vi "Driver Feedback Loop.vi"   [LabVIEW 2019]
uses:
  Shoot/Shooter Mode Type Def.ctl
  Shoot/Shoot Global.vi
  Vanna/Vanna Global.vi
  Vanna/Vanna Mode Type Def.ctl
  Drive/Drive Global.vi
  Drive/Drive Mode Typedef.ctl
types:
  T1 = typedef "WPI_MotorControlDeviceRef.ctl" = cluster{"DeviceStatus":errorcluster, "Type":T2, "PWM":cluster{"PWM Channel":T3, "DeadBand":T4}, "CAN":cluster{"Device Number":u8, "SetOutput VI Ref":variant, "GetOutput VI Ref":variant, "Enable VI Ref":variant, "Disable VI Ref":variant, "Data":variant}, "Invert":bool, "DIO PWM":cluster{"PWM \"Enable\" Channel":T3, "DIOChannel":T5, "PWM Rate":dbl}}
  T2 = typedef "WPI_MotorControlType.ctl" = enum16{"PWM", "CAN", "DIO PWM"}
  T3 = typedef "FPGA_DIOPWMChannel.ctl" = enum8{"PWM 0", "PWM 1", "PWM 2", "PWM 3", "PWM 4", "PWM 5", "PWM 6", "PWM 7", "PWM 8", "PWM 9", "PWM MXP 0", "PWM MXP 1", "PWM MXP 2", "PWM MXP 3", "PWM MXP 4", "PWM MXP 5", "PWM MXP 6", "PWM MXP 7", "PWM MXP 8", "PWM MXP 9", "Invalid"}
  T4 = typedef "WPI_PWMDeadband.ctl" = cluster{"Name":string, "maxPositivePwm":i32, "minPositivePwm":i32, "centerPwm":i32, "maxNegativePwm":i32, "minNegativePwm":i32, "angularRange":u16}
  T5 = typedef "FPGA_DIOChannel.ctl" = enum8{"DIO 0", "DIO 1", "DIO 2", "DIO 3", "DIO 4", "DIO 5", "DIO 6", "DIO 7", "DIO 8", "DIO 9", "DIO MXP 0", "DIO MXP 1", "DIO MXP 2", "DIO MXP 3", "DIO MXP 4", "DIO MXP 5", "DIO MXP 6", "DIO MXP 7", "DIO MXP 8", "DIO MXP 9", "DIO MXP 10", "DIO MXP 11", "DIO MXP 12", "DIO MXP 13", "DIO MXP 14", "DIO MXP 15", "SPI Port CS1", "SPI Port CS2", "SPI Port CS3", "SPI Port MISO", "SPI Port MOSI", "Invalid"}
  T6 = typedef "WPI_JoystickDevRef.ctl" = cluster{"Device":T7}
  T7 = typedef "WPI_JoystickDeviceEnum.ctl" = enum16{"USB 0", "USB 1", "USB 2", "USB 3", "USB 4", "USB 5"}
  T8 = typedef "Shooter Mode Type Def.ctl" = enum16{"Disabled", "Raw Throttle", "Preset Velocity Control", "Vision-based Velocity Control"}
  T9 = typedef "Drive Mode Typedef.ctl" = enum16{"Disabled", "Auto-align", "Drive Distance", "Turn to angle", "Driver"}
  T10 = typedef "Vanna Mode Type Def.ctl" = enum16{"Disabled", "Raw Throttle", "Rotation Control", "Position Control"}
  T11 = typedef "Vanna Command Type Def.ctl" = cluster{"Vanna Mode":T10, "Throttle (%)":dbl, "Timestamp (ms)":dbl}
  T12 = typedef "Drive Command Typedef.ctl" = cluster{"Drive Mode":T9, "LeftValue(%)/ relative Distance[ft]":dbl, "Right Motor Value(%)/ absolute angle (deg)":dbl, "Timestamp (ms)":dbl}
  T13 = typedef "Shooter Command Type Def.ctl" = cluster{"Shooter Mode":T8, "Throttle (%)/ Vision-based\nSetpoint (RPM)":dbl, "Shooter Preset speeds (RPM)":T14, "Timestamp (ms)":dbl}
  T14 = typedef "Shooter Preset speeds Type Def.ctl" = enum16{"Not Applicable", "Target Zone", "Initiation Line", "Close end of Trench Run", "Control Panel"}
  T15 = typedef "Is command done typedef.ctl" = cluster{"Done?":bool, "Timestamp [ms]":dbl}
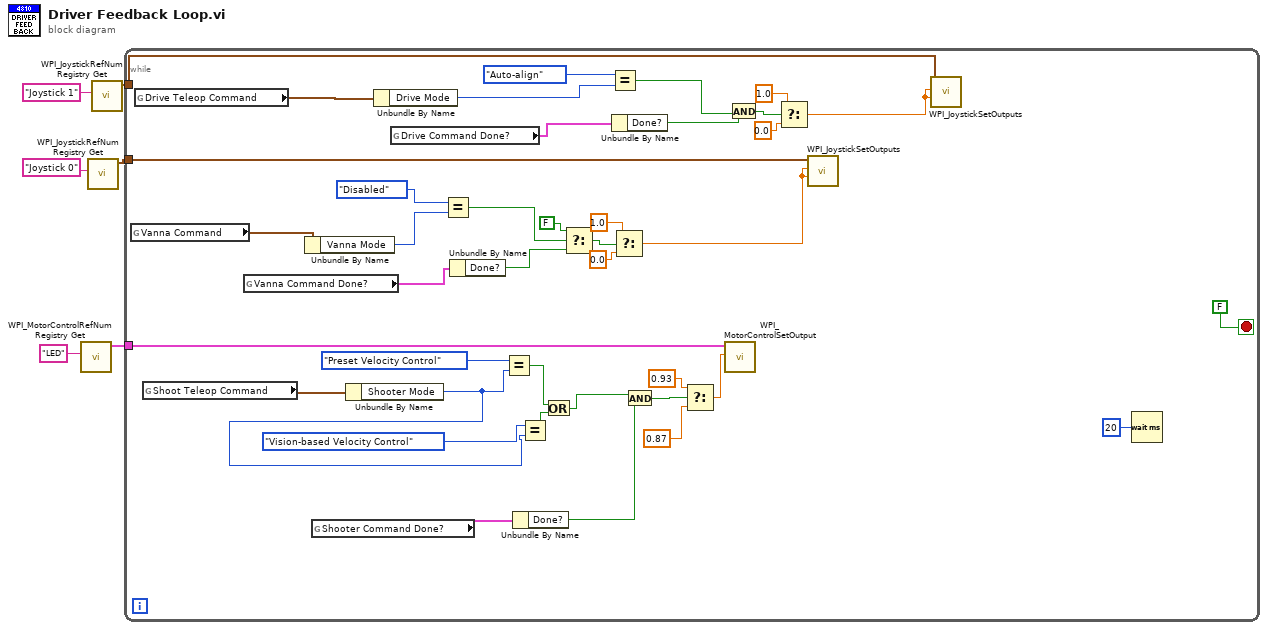
[diagram p0: block diagram]
diagram:
  n1 = call <vilib>:"WPI_MotorControlRefNum Registry Get.vi"("refnum name"="LED") -> ("MotorControlDevRef"=w1:T1)  [unwired: 9 in, 1 out]
  n2 = call <vilib>:"WPI_JoystickRefNum Registry Get.vi"("refnum name"="Joystick 0") -> ("JoystickDevRef"=w6:T6)  [unwired: 9 in, 1 out]
  n3 = call <vilib>:"WPI_JoystickRefNum Registry Get.vi"("refnum name"="Joystick 1") -> ("JoystickDevRef"=w5:T6)  [unwired: 9 in, 1 out]
  n4 = while {
    tunnel: w6 -> [w43]
    tunnel: w5 -> [w42]
    tunnel: w1 -> [w35]
    stop <- FALSE stop-if-true
    n5 = global read "Vanna Global.vi" "Vanna Command"() -> (w19:T11)
    n6 = global read "Drive Global.vi" "Drive Teleop Command"() -> (w16:T12)
    n7 = global read "Shoot Global.vi" "Shoot Teleop Command"() -> (w27:T13)
    n8 = global read "Vanna Global.vi" "Vanna Command Done?"() -> (w12:cluster{"Done?":bool, "Timestamp (ms)":dbl})
    n9 = Unbundle By Name(w19) -> ("Vanna Mode"=w18:T10)
    n10 = global read "Shoot Global.vi" "Shooter Command Done?"() -> (w40:T15)
    n11 = Unbundle By Name(w27) -> ("Shooter Mode"=w10:T8)
    n12 = Unbundle By Name(w16) -> ("Drive Mode"=w15:T9)
    n13 = global read "Drive Global.vi" "Drive Command Done?"() -> (w13:T15)
    n14 = Equal?(x=Vanna_Mode_Type_Def."Disabled" ("Vanna Mode"), y=w18) -> (x = y?=w26:bool)
    n15 = Unbundle By Name(w12) -> ("Done?"=w25:bool)
    n16 = Equal?(x=Shooter_Mode_Type_Def."Preset Velocity Control" ("Shooter Mode"), y=w10) -> (x = y?=w9:bool)
    n17 = Unbundle By Name(w40) -> ("Done?"=w39:bool)
    n18 = Equal?(x=Shooter_Mode_Type_Def."Vision-based Velocity Control" ("Shooter Mode"), y=w10) -> (x = y?=w8:bool)
    n19 = Or(x=w9, y=w8) -> (x .or. y?=w7:bool)
    n20 = Select(t=FALSE, s=w26, f=w25) -> (s? t:f=w24:bool)
    n21 = Equal?(x=Drive_Mode_Typedef."Auto-align" ("Drive Mode"), y=w15) -> (x = y?=w33:bool)
    n22 = Unbundle By Name(w13) -> ("Done?"=w32:bool)
    n23 = Select(t=sgl 1.0 ("Left Rumble"), s=w24, f=sgl 0.0 ("Left Rumble")) -> (s? t:f=w20:sgl)
    n24 = And(x=w7, y=w39) -> (x .and. y?=w38:bool)
    n25 = Select(t=0.93, s=w38, f=0.87) -> (s? t:f=w34:dbl)
    n26 = call <vilib>:"WPI_MotorControlSetOutput.vi"("Output"=w34, "MotorControlDevRef"=w35) -> ()  [unwired: 7 in, 3 out]
    n27 = And(x=w33, y=w32) -> (x .and. y?=w30:bool)
    n28 = Select(t=sgl 1.0 ("Left Rumble"), s=w30, f=sgl 0.0 ("Left Rumble")) -> (s? t:f=w28:sgl)
    n29 = call <vilib>:"WPI_JoystickSetOutputs.vi"("Right Rumble"=w20, "Left Rumble"=w20, "JoystickDevRef"=w43) -> ()  [unwired: 7 in, 2 out]
    n30 = call <vilib>:"WPI_JoystickSetOutputs.vi"("Right Rumble"=w28, "Left Rumble"=w28, "JoystickDevRef"=w42) -> ()  [unwired: 7 in, 2 out]
    n31 = Wait (ms)(milliseconds to wait=u32 20 ("millisecond timer value")) -> ()  [unwired: 1 out]
  }
